vi "Test 10-Tap 8-bit Camera with DRAM (FPGA).vi"() -> ()   [LabVIEW 2013]
doc: "This is the FPGA VI for the 10-Tap 8-Bit Camera with DRAM example. This example demonstrates how to acquire images from a 10-tap, 8-bit, extended configuration, Camera Link camera and transfer the images to the host. This example supports area scan and line scan cameras for both continuous and finite acquisitions.\n\nThis example also demonstrates the use of DRAM as a frame buffer for very high speed acquisitions. Data packing and flow-control are also employed to maximize use of the available DRAM and FIFOs in terms of both memory space and performance.\n\nAdditionally, the example demonstrates the serial server, which allows third-party camera configuration utilities to communicate with the camera using the Camera Link serial interface while this VI is running."
uses:
  <vilib>/rvi/DataTransferAndStorage/Container/XNode/niFpgaContainer.xnode
  <vilib>/Platform/TimedLoop/XDataNode/XDataNode.xnode
  <vilib>/Platform/TimedLoop/XDataNode/timing_clust.ctl
  <vilib>/Platform/TimedLoop/XDataNode/XDNodeRunTimeDep.lvlib
  <vilib>/Platform/TimedLoop/XDataNode/wakeup.ctl
  <vilib>/Platform/TimedLoop/XDataNode/nitl_modes.ctl
  <vilib>/eio/EIONode/EIONode.xnode
  <vilib>/rvi/eio/common/nirviEmuTemplateMethod_errors.vi
  <vilib>/rvi/FIFO/Fifo_Resource/nirvififoEmulationGetNumberOfElementsToRead.vi
  <vilib>/rvi/interface/RandomDataEmulation/nirviRandomDataFpgaReadWriteTemplate.vi
  <vilib>/rvi/FIFO/Fifo_Resource/nirvififoEmulationRead.vi
  <vilib>/rvi/FIFO/Fifo_Resource/nirvififoEmulationWrite.vi
  Common/CL Data to Pixels/10 Tap 8-Bit.vi
  FPGA/10-Tap Data/10-Tap Conversion Enum.ctl
  FPGA/Globals/Accumulated Sector Intensity.vi
  FPGA/Globals/Pixel Location Global.vi
  FPGA/Globals/Wing Square Wave Frequency Global.vi
  <vilib>/rvi/FIFO/Fifo_Resource/nirvififoEmulationGetNumberOfElementsToWrite.vi
  Common/CL Signal Mapping.ctl
  Common/CL Configuration.ctl
  FPGA/Sector/Accumulate/Sector Parameter Cluster.ctl
panel:
  in  "Sector Threshold":u8
  in  "# of Frames to Average":u8
  in  "Sector Parameters Right":T1={"Start Angle"=0.13543701171875, "End Angle"=0.30462646484375, "Inner Radius"=309, "Outter Radius"=405, "Hinge X"=1106, "Hinge Y"=803, "NumWingSectors"=8}
  in  "Sector Parameters Left":T1={"Start Angle"=0.6541748046875, "End Angle"=0.856201171875, "Inner Radius"=309, "Outter Radius"=405, "Hinge X"=947, "Hinge Y"=829, "NumWingSectors"=8}
  in  "Sim":bool=TRUE
  in  "CL Config.Configuration":T2=enum."Full"
  in  "CL Config.Signal Mapping":T3=enum."Basler 10-tap"
  in  "CL Config.Line Scan":bool
  in  "CL Config.DVAL Active High":bool=TRUE
  in  "CL Config.LVAL Active High":bool=TRUE
  in  "CL Config.FVAL Active High":bool=TRUE
  in  "CL Config.Spare Active High":bool=TRUE
  in  "Acq Control.Line Scan Height":u32
  in  "Acq Control.Frames To Acq":u32
  in  "Acq Control.Acquire":bool
  in  "Acq Control.Cancel Acq":bool
  in  "Acq Control.Ignore DVAL":bool
  in  "Acq Control.Initialize":bool
  out "Acq Status.Acq In Progress":bool
  out "Acq Status.Clocks Per Line":u32
  out "Acq Status.Frames Acq'd":u32
  out "Acq Status.Lines Per Frame":u32
  out "Acq Status.DMA Write Timeout":bool
  out "Acq Status.Initialized":bool
  in  "UART.Baud Rate":u8
  in  "UART.Transmit":bool
  in  "UART.Tx Data":u8[](array[numeric])=[0, 0, 0, 0, 0, 0, 0, 0, 0, 0] format="%02x"
  in  "UART.Set Baud Rate":bool
  in  "UART.Byte Mode":bool=TRUE
  out "UART.Rx Ready":bool
  out "UART.Break Indicator":bool
  out "UART.Framing Error":bool
  out "UART.Overrun Error":bool
  out "UART.Tx Ready":bool
  out "UART.Rx Data":u8 format="%02x"
  in  "UART.Receive":bool
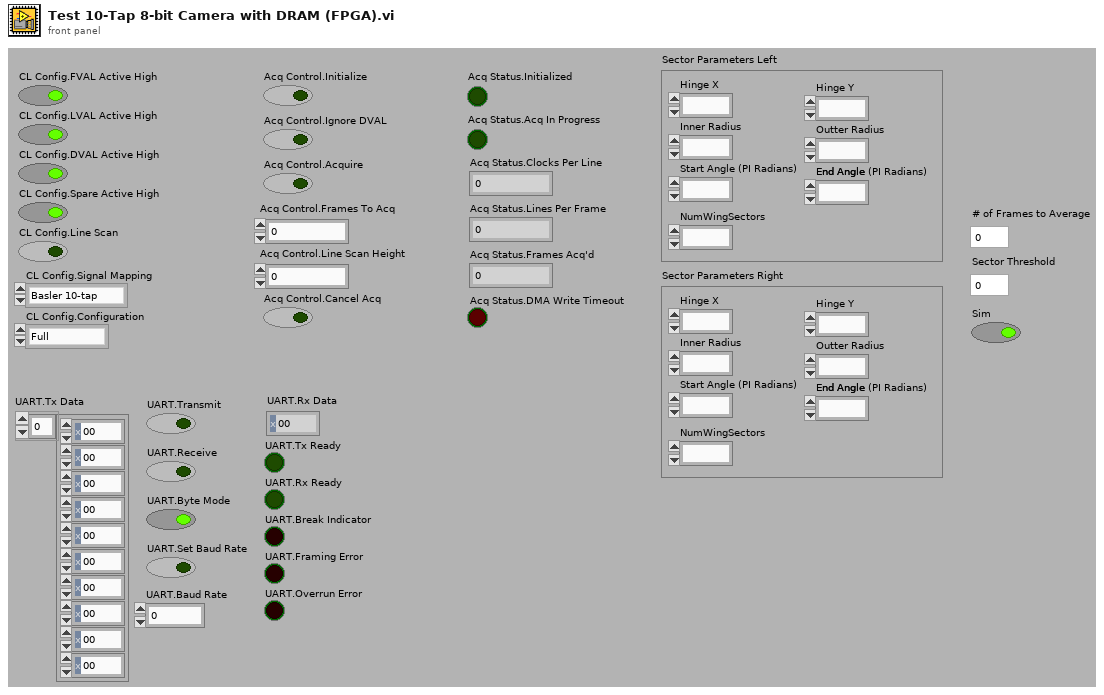
[diagram p1: front panel]
types:
  T1 = typedef "Sector Parameter Cluster.ctl" = cluster{"Start Angle":fxp<+/-,17,2>, "End Angle":fxp<+,17,3>, "Inner Radius":u16, "Outter Radius":u16, "Hinge X":u16, "Hinge Y":u16, "NumWingSectors":u8}
  T2 = typedef "CL Configuration.ctl" = enum8{"Base", "Medium", "Full"}
  T3 = typedef "CL Signal Mapping.ctl" = enum8{"Standard", "Basler 10-tap", "Vosskühler 10-tap"}
  T4 = typedef "XDNodeRunTimeDep.lvlib/timing_clust.ctl" = cluster{"Expected End [f-1]":u64, "Actual End [f-1]":u64, "Finished Late? [f-1]":bool, "Expected End [i-1]":u64, "Actual End [i-1]":u64, "Finished Late? [i-1]":bool, "Expected Start [i]":u64, "Actual Start [i]":u64, "Expected Start [f]":u64, "Actual Start [f]":u64, "Source Name":string, "Structure Name":string, "Period":i64, "Deadline":i64, "Offset":i64, "Start":i64, "Priority":i32, "Timeout":i32, "Mode":T5, "Wakeup Reason":T6, "Error":errorcluster, "Source Type":string, "Secondary Source Type":string, "Global End Time":u64, "Global Start Time":u64, "Frame Duration":u64, "Iteration Duration":u64, "Assigned CPU":i32, "I/O Scan Engine Mode":u32}
  T5 = typedef "XDNodeRunTimeDep.lvlib/nitl_modes.ctl" = enum32{"No Change", "Process missed periods, maintain original phase", "Discard missed periods, maintain original phase", "Process missed periods, ignore original phase", "Discard missed periods, ignore original phase"}
  T6 = typedef "XDNodeRunTimeDep.lvlib/wakeup.ctl" = enum32{"Normal", "Aborted", "Asynchronous wakeup", "Timing source error", "Timed loop error", "Timeout"}
  T7 = typedef "10-Tap Conversion Enum.ctl" = enum16{"10-Tap to 16 and 64", "16 and 64 to 10-Tap"}
  T8 = cluster{"Enables Valid":bool, "Frame Valid":bool, "Line Valid":bool, "Data Valid":bool}
  T9 = typedef "10-Tap 8-bit Cluster.ctl" = cluster{"Pixel 0":u8, "Pixel 1":u8, "Pixel 2":u8, "Pixel 3":u8, "Pixel 4":u8, "Pixel 5":u8, "Pixel 6":u8, "Pixel 7":u8, "Pixel 8":u8, "Pixel 9":u8}
  T10 = cluster{"Tx Data":u8[], "Transmit":bool, "Receive":bool, "Byte Mode":bool, "Set Baud Rate":bool, "Baud Rate":u8}
  T11 = cluster{"Rx Data":u8, "Turn Off Transmit":bool, "Turn Off Receive":bool, "Turn Off Set Baud Rate":bool, "Tx Ready":bool, "Rx Ready":bool, "Break Indicator":bool, "Framing Error":bool, "Overrun Error":bool}
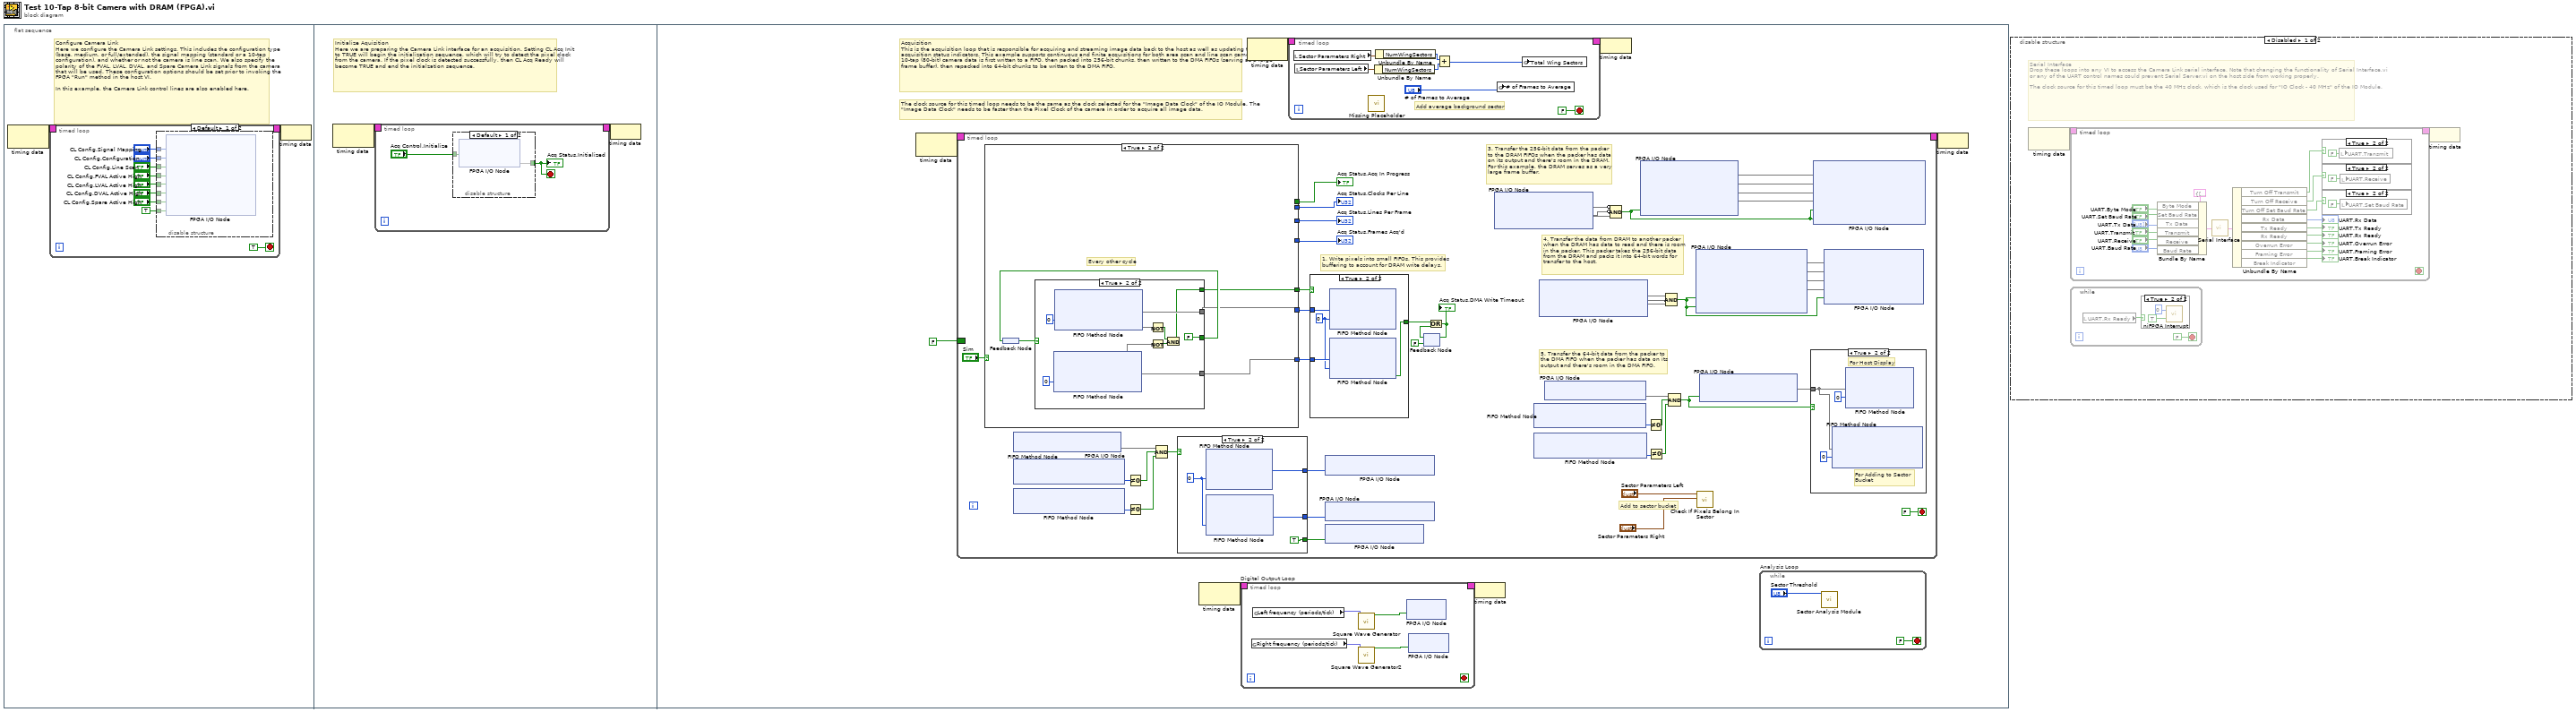
[diagram p0: block diagram]
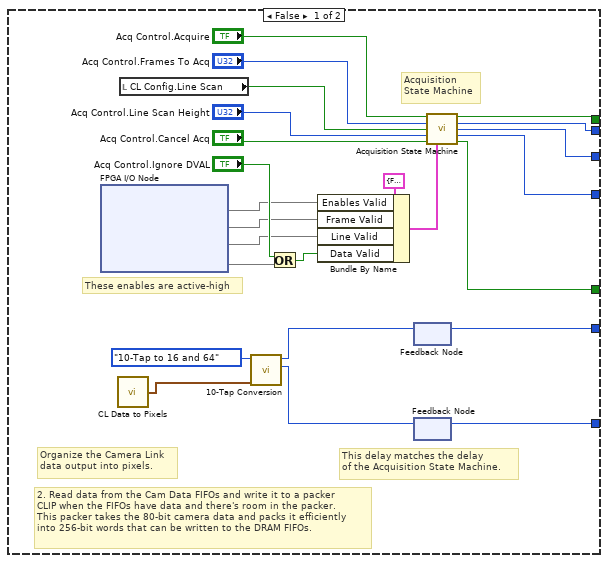
[diagram p10: hidden frame]
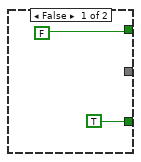
[diagram p11: hidden frame]
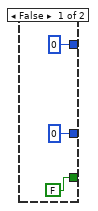
[diagram p12: hidden frame]
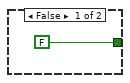
[diagram p13: hidden frame]
diagram:
  n1 = flat-sequence {
    frame #0 {
      # "Configure Camera Link\nHere we configure the Camera Link settings. This includes the configuration type (base, medium, or full/extended), the signal mapping (standard or a 10-tap configuration), and whether or not the camera is line scan. We also specify the polarity of the FVAL, LVAL, DVAL, and Spare Camera Link signals from the camera that will be used. These configuration options should be set prior to invoking the FPGA \"Run\" method in the host VI.\n\nIn this example, the Camera Link control lines are also enabled here."
      n2 = node-c288() -> (w2:T4)  [unwired: 1 in]
      n3 = timed-loop {
        timing: w2 -> [_]
        timing-out: [_] -> w1
        stop <- TRUE stop-if-true
        n4 = disable-structure shown="Default" {
          disable-tunnel: "CL Config.FVAL Active High" -> [w19 _]
          disable-tunnel: "CL Config.LVAL Active High" -> [w18 _]
          disable-tunnel: "CL Config.DVAL Active High" -> [w17 _]
          disable-tunnel: "CL Config.Spare Active High" -> [w16 _]
          disable-tunnel: "CL Config.Signal Mapping" -> [w15 _]
          disable-tunnel: "CL Config.Configuration" -> [w14 _]
          disable-tunnel: "CL Config.Line Scan" -> [w13 _]
          disable-tunnel: TRUE ("IO Module\\CL Control Enable") -> [w12 _]
          frame condition #0 {
            n5 = xnode "FPGA I/O Node"("CL Set Signal Mapping"=w15, "CL Set Configuration"=w14, "CL Set Line Scan"=w13, "CL Set FVAL Active High"=w19, "CL Set LVAL Active High"=w18, "CL Set DVAL Active High"=w17, "CL Set Spare Active High"=w16, "CL Control Enable"=w12) -> ()  [unwired: 8 in, 8 out]
          }
          frame condition #1 (active) {
          }
        }
      }
      n6 = node-c288(w1) -> ()
    }
    frame #1 {
      # "Initialize Aquisition\nHere we are preparing the Camera Link interface for an acquisition. Setting CL Acq Init to TRUE will begin the initialization sequence, which will try to detect the pixel clock from the camera. If the pixel clock is detected successfully, then CL Acq Ready will become TRUE and end the initialzation sequence."
      n7 = node-c288() -> (w25:T4)  [unwired: 1 out]
      n8 = timed-loop {
        timing: w25 -> [_]
        timing-out: [_] -> w24
        stop <- w26 stop-if-true
        n9 = disable-structure shown="Default" {
          disable-tunnel: "Acq Control.Initialize" -> [w29 w30]
          disable-tunnel: [w28 w30] -> w26
          frame condition #0 {
            n10 = xnode "FPGA I/O Node"("CL Acq Init"=w29) -> ("CL Acq Ready"=w28)  [unwired: 2 in, 2 out]
          }
          frame condition #1 (active) {
          }
        }
        "Acq Status.Initialized" <- w26
      }
      n11 = node-c288(w24) -> ()
    }
    frame #2 {
      # "The clock source for this timed loop needs to be the same as the clock selected for the \"Image Data Clock\" of the IO Module. The \"Image Data Clock\" needs to be faster than the Pixel Clock of the camera in order to acquire all image data."
      # "Acquisition\nThis is the acquisition loop that is responsible for acquiring and streaming image data back to the host as well as updating the acquisition status indicators. This example supports continuous and finite acquisitions for both area scan and line scan cameras. The 10-tap (80-bit) camera data is first written to a FIFO, then packed into 256-bit chunks, then written to the DMA FIFOs (serving as a large frame buffer), then repacked into 64-bit chunks to be written to the DMA FIFO."
      n12 = node-c288() -> (w41:T4)  [unwired: 1 in]
      n13 = timed-loop {
        timing: w41 -> [_]
        timing-out: [_] -> w40
        border: FALSE -> [_]
        stop <- FALSE stop-if-true
        # "Add to sector bucket"
        # "5. Transfer the 64-bit data from the packer to\nthe DMA FIFO when the packer has data on its\noutput and there's room in the DMA FIFO."
        # "4. Transfer the data from DRAM to another packer\nwhen the DRAM has data to read and there is room\nin the packer. This packer takes the 256-bit data\nfrom the DRAM and packs it into 64-bit words for\ntransfer to the host."
        # "3. Transfer the 256-bit data from the packer\nto the DRAM FIFOs when the packer has data\non its output and there's room in the DRAM.\nFor this example, the DRAM serves as a very\nlarge frame buffer."
        # "1. Write pixels into small FIFOs. This provides\nbuffering to account for DRAM write delays."
        n14 = case shown="True" "Sim" {
          tunnel: [w135 w136] -> w108
          tunnel: [w134 w137] -> w103
          tunnel: [w116 w139] -> w91
          tunnel: [w120 _] -> w90
          tunnel: [w119 _] -> w89
          tunnel: [w118 _] -> w88
          tunnel: [w117 _] -> w87
          frame False {
            # "These enables are active-high"
            # "Acquisition\nState Machine"
            # "2. Read data from the Cam Data FIFOs and write it to a packer\nCLIP when the FIFOs have data and there's room in the packer.\nThis packer takes the 80-bit camera data and packs it efficiently\ninto 256-bit words that can be written to the DRAM FIFOs."
            # "Organize the Camera Link\ndata output into pixels."
            # "This delay matches the delay\nof the Acquisition State Machine."
            n15 = xnode "FPGA I/O Node"() -> ("CL Output Valid"=w124, "CL Frame Valid"=w125, "CL Line Valid"=w126, "CL Data Valid"=w129)  [unwired: 4 in, 4 out]
            n16 = call-poly "CL Data to Pixels.vi"() -> ("Pixels"=w112:T9)  [unwired: 1 in]
            n17 = local read "CL Config.Line Scan"() -> (w132:bool)
            n18 = call "10-Tap Conversion.vi"("10 Tap In"=w112, "Operation"=10-Tap_Conversion_Enum."10-Tap to 16 and 64") -> ("64 Bit Out"=w113:u64, "16 Bit Out"=w114:u16)  [unwired: 7 in, 1 out]
            n19 = Or(x="Acq Control.Ignore DVAL", y=w129) -> (x .or. y?=w130:bool)
            n20 = Bundle By Name(cluster=T8 {"Enables Valid"=FALSE, "Frame Valid"=FALSE, "Line Valid"=FALSE, "Data Valid"=FALSE} ("Enables"), "Enables Valid"=w124, "Frame Valid"=w125, "Line Valid"=w126, "Data Valid"=w130) -> (w127:T8)
            n21 = feedback #1() -> (w134:u16)  [unwired: 1 in]
            n22 = feedback-in #1(w114) -> ()
            n23 = feedback #2() -> (w135:u64)  [unwired: 1 in]
            n24 = feedback-in #2(w113) -> ()
            n25 = call "Acquisition State Machine.vi"("Acquire"="Acq Control.Acquire", "Frames to Acquire"="Acq Control.Frames To Acq", "Line Scan"=w132, "Line Scan Height"="Acq Control.Line Scan Height", "Cancel Acq"="Acq Control.Cancel Acq", "Enables"=w127) -> ("Acq In Progress"=w120:bool, "Num Clocks Per Line"=w119:u32, "Num Lines Per Frame"=w118:u32, "Num Frames Acq'd"=w117:u32, "Capture Cycle"=w116:bool)  [unwired: 4 in, 1 out]
          }
          frame True {
            # "Every other cycle"
            n26 = feedback #3() -> (w138:bool)
            n27 = case shown="True" w138 {
              tunnel: [_ w152] -> w137
              tunnel: [_ w151] -> w136
              tunnel: [FALSE w144] -> w139
              tunnel: [TRUE FALSE] -> w140
              frame False {
              }
              frame True {
                n28 = xnode ("FIFO Method Node")("Timeout"=0) -> ("Element"=w151, "Timed Out?"=w147)  [unwired: 1 in, 1 out]
                n29 = xnode ("FIFO Method Node")("Timeout"=0) -> ("Element"=w152, "Timed Out?"=w148)  [unwired: 1 in, 1 out]
                n30 = Not(x=w148) -> (.not. x?=w146:bool)
                n31 = Not(x=w147) -> (.not. x?=w145:bool)
                n32 = And(x=w146, y=w145) -> (x .and. y?=w144:bool)
              }
            }
            n33 = feedback-in #3(w140) -> ()
          }
        }
        "Acq Status.Frames Acq'd" <- w87
        "Acq Status.Lines Per Frame" <- w88
        "Acq Status.Clocks Per Line" <- w89
        "Acq Status.Acq In Progress" <- w90
        n34 = xnode "FPGA I/O Node"() -> ("Pack 80 to 256\\Ready For Write"=w97)  [unwired: 1 in, 1 out]
        n35 = xnode ("FIFO Method Node")() -> ("Number of Elements to Read"=w101:u32)  [unwired: 1 in, 1 out]
        n36 = xnode ("FIFO Method Node")() -> ("Number of Elements to Read"=w100:u32)  [unwired: 1 in, 1 out]
        n37 = Not Equal To 0?(x=w101) -> (x != 0?=w95:bool)
        n38 = Not Equal To 0?(x=w100) -> (x != 0?=w94:bool)
        n39 = Compound Arithmetic op=AND(w97, w95, w94) -> (w96:bool)
        n40 = case shown="True" w96 {
          tunnel: [u16 0 ("Element") w159] -> w102
          tunnel: [u64 0 ("Element") w158] -> w98
          tunnel: [FALSE TRUE] -> w99
          frame False {
          }
          frame True {
            w157 = 0 ("Timeout")
            n41 = xnode ("FIFO Method Node")("Timeout"=w157) -> ("Element"=w159:u16)  [unwired: 1 in, 2 out]
            n42 = xnode ("FIFO Method Node")("Timeout"=w157) -> ("Element"=w158:u64)  [unwired: 1 in, 2 out]
          }
        }
        n43 = case shown="True" w91 {
          tunnel: [FALSE ("Timed Out?") w163] -> w106
          tunnel: w108 -> [_ w164]
          tunnel: w103 -> [_ w162]
          frame False {
          }
          frame True {
            w161 = 0 ("Timeout")
            n44 = xnode ("FIFO Method Node")("Element"=w162, "Timeout"=w161) -> ()  [unwired: 1 in, 2 out]
            n45 = xnode ("FIFO Method Node")("Element"=w164, "Timeout"=w161) -> ("Timed Out?"=w163:bool)  [unwired: 1 in, 1 out]
          }
        }
        n46 = xnode "FPGA I/O Node"("Pack 80 to 256\\Data In Upper 16"=w102) -> ()  [unwired: 1 in, 1 out]
        n47 = xnode "FPGA I/O Node"("Pack 80 to 256\\Data In Lower 64"=w98) -> ()  [unwired: 1 in, 1 out]
        n48 = xnode "FPGA I/O Node"("Pack 80 to 256\\Write Enable"=w99) -> ()  [unwired: 1 in, 1 out]
        n49 = feedback #4(FALSE) -> (w105:bool)
        n50 = Or(x=w106, y=w105) -> (x .or. y?=w104:bool)
        "Acq Status.DMA Write Timeout" <- w104
        n51 = feedback-in #4(w104) -> ()
        n52 = xnode "FPGA I/O Node"() -> ("DRAM Bank 0\\Full"=w67, "Pack 80 to 256\\Output Valid"=w86)  [unwired: 3 in, 4 out]
        n53 = xnode ("FIFO Method Node")() -> ("Number of Elements to Write"=w69:u32)  [unwired: 1 in, 1 out]
        n54 = xnode ("FIFO Method Node")() -> ("Number of Elements to Write"=w66:u32)  [unwired: 1 in, 1 out]
        n55 = xnode "FPGA I/O Node"() -> ("DRAM Bank 1\\Data_Available"=w80, "DRAM Bank 0\\Data_Available"=w78, "Pack 256 To 64\\Ready for Write"=w79)  [unwired: 3 in, 3 out]
        n56 = xnode "FPGA I/O Node"() -> ("Pack 256 To 64\\Output Valid"=w71)  [unwired: 1 in, 1 out]
        n57 = Compound Arithmetic op=AND(invert w67, invert w67, w86) -> (w81:bool)
        n58 = xnode "FPGA I/O Node"("Pack 80 to 256\\Read Enable"=w81) -> ("Pack 80 To 256\\Data Out 3"=w85, "Pack 80 To 256\\Data Out 2"=w84, "Pack 80 To 256\\Data Out 1"=w83, "Pack 80 To 256\\Data Out 0"=w82)  [unwired: 5 in, 5 out]
        n59 = Not Equal To 0?(x=w69) -> (x != 0?=w70:bool)
        n60 = Not Equal To 0?(x=w66) -> (x != 0?=w65:bool)
        n61 = Compound Arithmetic op=AND(w80, w78, w79) -> (w73:bool)
        n62 = Compound Arithmetic op=AND(w71, w70, w65) -> (w68:bool)
        n63 = xnode "FPGA I/O Node"("DRAM Bank 1\\Read"=w73, "DRAM Bank 0\\Read"=w73) -> ("DRAM Bank 1\\Read_Data_Upper"=w77, "DRAM Bank 1\\Read_Data_Lower"=w76, "DRAM Bank 0\\Read_Data_Upper"=w75, "DRAM Bank 0\\Read_Data_Lower"=w74)  [unwired: 6 in, 6 out]
        n64 = call "Check If Pixels Belong In Sector.vi"(10:"Sector Parameters Right", 11:"Sector Parameters Left") -> ()  [unwired: 9 in, 1 out]
        n65 = xnode "FPGA I/O Node"("Pack 256 to 64\\Read Enable"=w68) -> ("Pack 256 To 64\\Data Out 64"=w72)  [unwired: 2 in, 2 out]
        n66 = case shown="True" w68 {
          tunnel: w72 -> [_ w110]
          frame False {
          }
          frame True {
            # "For Adding to Sector \nBucket"
            # "For Host Display"
            n67 = xnode ("FIFO Method Node")("Element"=w110, "Timeout"=0) -> ()  [unwired: 1 in, 2 out]
            n68 = xnode ("FIFO Method Node")("Element"=w110, "Timeout"=0) -> ()  [unwired: 1 in, 2 out]
          }
        }
        n69 = xnode "FPGA I/O Node"("DRAM Bank 1\\Write_Data_Upper"=w85, "DRAM Bank 1\\Write_Data_Lower"=w84, "DRAM Bank 0\\Write_Data_Upper"=w83, "DRAM Bank 0\\Write_Data_Lower"=w82, "DRAM Bank 1\\Write"=w81, "DRAM Bank 0\\Write"=w81) -> ()  [unwired: 6 in, 6 out]
        n70 = xnode "FPGA I/O Node"("Pack 256 To 64\\Data In 3"=w77, "Pack 256 To 64\\Data In 2"=w76, "Pack 256 To 64\\Data In 1"=w75, "Pack 256 To 64\\Data In 0"=w74, "Pack 256 to 64\\Write Enable"=w73) -> ()  [unwired: 5 in, 5 out]
      }
      n71 = node-c288() -> (w38:T4)  [unwired: 1 in]
      n72 = timed-loop "Digital Output Loop" {
        timing: w38 -> [_]
        timing-out: [_] -> w37
        stop <- _ stop-if-true
        n73 = global read "Wing Square Wave Frequency Global.vi" "Right frequency (periods/tick)"() -> (w55:fxp<+,32,0>)
        n74 = global read "Wing Square Wave Frequency Global.vi" "Left frequency (periods/tick)"() -> (w56:fxp<+,32,0>)
        n75 = call "Square Wave Generator"("frequency (periods/tick)"=w56) -> ("square wave out"=w58:bool)  [unwired: 14 in]
        n76 = call "Square Wave Generator2"("frequency (periods/tick)"=w55) -> ("square wave out"=w57:bool)  [unwired: 14 in]
        n77 = xnode "FPGA I/O Node"("TTL 0"=w58) -> ()  [unwired: 1 in, 1 out]
        n78 = xnode "FPGA I/O Node"("TTL 1"=w57) -> ()  [unwired: 1 in, 1 out]
      }
      n79 = node-c288() -> (w36:T4)  [unwired: 1 in]
      n80 = timed-loop {
        timing: w36 -> [_]
        timing-out: [_] -> w35
        stop <- FALSE stop-if-true
        # "Add average background sector"
        n81 = local read "Sector Parameters Right"() -> (w47:T1)
        n82 = local read "Sector Parameters Left"() -> (w46:T1)
        n83 = call "Missing Placeholder.vi"() -> ()  [unwired: 12 in]
        n84 = Unbundle By Name(w46) -> ("NumWingSectors"=w44:u8)
        n85 = Unbundle By Name(w47) -> ("NumWingSectors"=w45:u8)
        n86 = Add(x=w45, y=w44) -> (x+y=w43:u8)
        n87 = global write "Pixel Location Global.vi" "# of Frames to Average"("# of Frames to Average") -> ()
        n88 = global write "Accumulated Sector Intensity.vi" "Total Wing Sectors"(w43) -> ()
      }
      n89 = node-c288(w37) -> ()
      n90 = node-c288(w35) -> ()
      n91 = while "Analysis Loop" {
        stop <- FALSE stop-if-true
        n92 = call "Sector Analysis Module.vi"("Canceled?"="Sector Threshold") -> ()  [unwired: 6 in, 5 out]
      }
      n93 = node-c288(w40) -> ()
    }
  }
  n94 = disable-structure shown="Disabled" {
    frame Disabled {
      # "Serial Interface\nDrop these loops into any VI to access the Camera Link serial interface. Note that changing the functionality of Serial Interface.vi or any of the UART control names could prevent Serial Server.vi on the host side from working properly.\n\nThe clock source for this timed loop must be the 40 MHz clock, which is the clock used for \"IO Clock - 40 MHz\" of the IO Module."
      n95 = node-c288() -> (w170:T4)  [unwired: 1 out]
      n96 = timed-loop {
        timing: w170 -> [_]
        timing-out: [_] -> w169
        stop <- _ stop-if-true
        n97 = Bundle By Name(cluster=T10 {"Tx Data"=[0, 0, 0, 0, 0, 0, 0, 0, 0, 0], "Transmit"=FALSE, "Receive"=FALSE, "Byte Mode"=TRUE, "Set Baud Rate"=FALSE, "Baud Rate"=0} ("UART Inputs"), "Byte Mode"="UART.Byte Mode", "Set Baud Rate"="UART.Set Baud Rate", "Tx Data"="UART.Tx Data", "Transmit"="UART.Transmit", "Receive"="UART.Receive", "Baud Rate"="UART.Baud Rate") -> (w175:T10)
        n98 = call "Serial Interface.vi"("UART Inputs"=w175) -> ("UART Outputs"=w187:T11)
        n99 = Unbundle By Name(w187) -> ("Turn Off Transmit"=w180:bool, "Turn Off Receive"=w181:bool, "Turn Off Set Baud Rate"=w177:bool, "Rx Data"=→"UART.Rx Data":u8, "Tx Ready"=→"UART.Tx Ready":bool, "Rx Ready"=→"UART.Rx Ready":bool, "Overrun Error"=→"UART.Overrun Error":bool, "Framing Error"=→"UART.Framing Error":bool, "Break Indicator"=→"UART.Break Indicator":bool)
        n100 = case shown="True" w180 {
          frame False {
          }
          frame True {
            n101 = local write "UART.Transmit"(FALSE ("UART.Transmit")) -> ()
          }
        }
        n102 = case shown="True" w181 {
          frame False {
          }
          frame True {
            n103 = local write "UART.Receive"(FALSE ("UART.Receive")) -> ()
          }
        }
        n104 = case shown="True" w177 {
          frame False {
          }
          frame True {
            n105 = local write "UART.Set Baud Rate"(FALSE ("UART.Receive")) -> ()
          }
        }
      }
      n106 = while {
        stop <- FALSE stop-if-true
        n107 = local read "UART.Rx Ready"() -> (w172:bool)
        n108 = case shown="True" w172 {
          frame False {
          }
          frame True {
            n109 = call <vilib>:"niFPGA Interrupt.vi"("Wait Until Cleared (F)"=TRUE ("Wait Until Cleared"), "IRQ Number (0)"=u8 0 ("IRQ Number")) -> ()  [unwired: 1 in]
          }
        }
      }
      n110 = node-c288(w169) -> ()
    }
    frame Enabled {
    }
  }
